vi "TestRun.vi"() -> ()   [LabVIEW 2018, in "FgenPlugins.lvlib" / "DaqMx_Single.lvclass"]
uses:
  DaqMx_Single.lvclass
  X:/Projects/PMUCal/Modules/FGen/FgenPlugins/NiPxi6733Class/NiPxi6733.lvclass
  NiPxi6733Class/NiPxi6733.lvclass/NiPxi6733.ctl
  NiPxi6733Class/Accessors/Write SampleRate.vi
panel:
  out "error out":errorcluster
  in  "Stop Button":bool
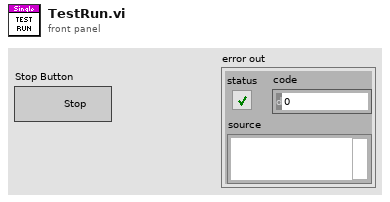
[diagram p1: front panel]
types:
  T1 = typedef "FgenPlugins.lvlib/DaqMx_Single.lvclass/clEvents.ctl" = cluster{"Stop":refnum<user-event>, "Params":refnum<user-event>}
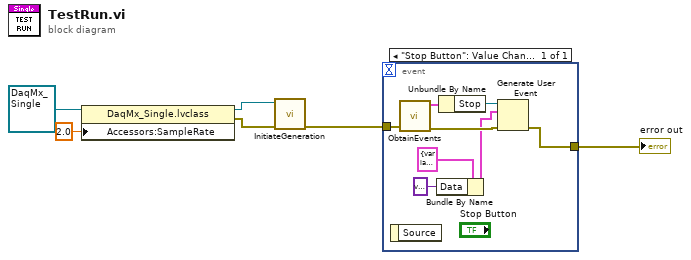
[diagram p0: block diagram]
diagram:
  n1 = property class="DaqMx_Single.lvclass"(reference=refnum<class "DaqMx_Single.lvclass"> refnum ("FgenPlugins.lvlib:DaqMx_Single.lvclass"), "Accessors:SampleRate"=2.0 ("SampleRate")) -> (reference out=w1:refnum<class "DaqMx_Single.lvclass">, error out=w2:errorcluster)  [unwired: 1 in]
  n2 = call-dynamic "InitiateGeneration.vi"("error in (no error)"=w2, "DaqMx_Single in"=w1) -> ("error out"=w3:errorcluster)  [unwired: 8 in, 1 out]
  n3 = event shown="[0] \"Stop Button\": Value Change" {
    selector: _ -> [_]
    dyn-events: _ -> [_]
    timeout: _ -> [_]
    tunnel: w3 -> [w14]
    tunnel: [w10] -> w6
    event "Stop Button": Value Change {
      n4 = event-data() -> ()  [unwired: 1 in, 1 out]
      n5 = call "ObtainEvents.vi"("error in (no error)"=w14) -> ("error out"=w11:errorcluster, "clEvent"=w13:T1)  [unwired: 9 in]
      n6 = Bundle By Name(cluster=cluster{"Data":variant} {"Data"=variant} ("event data"), "Data"=variant) -> (w8:cluster{"Data":variant})
      n7 = Unbundle By Name(w13) -> ("Stop"=w12:refnum<user-event>)
      n8 = Generate User Event(user event=w12, event data cluster=w8, error in=w11) -> (error out=w10:errorcluster)  [unwired: 1 in, 1 out]
    }
  }
  "error out" <- w6
